vi "CreateQueueName.vi"(0 "VI reference in":refnum<vi> caption="VI reference in (Top-Level)", 11 "Error in":errorcluster caption="Error in (no error)") -> (4 "Queue name":string, 15 "Error out":errorcluster)   [LabVIEW 2017, in "VILauncher.lvlib"]
doc: "Creates the <B>Queue name</B> for the AutoQueue used by the DynamicDispatch toolset.\n\nThis VI is reentrant, and it doesn't run if there is an error on <B>Error in</B>.\n\nSteen Schmidt\nGPower\n26/12 2012"
uses:
  VILauncher.lvlib
panel:
  # "Copyright © 2013\nSteen Schmidt, GPower\nSee enclosed license file for terms and conditions"
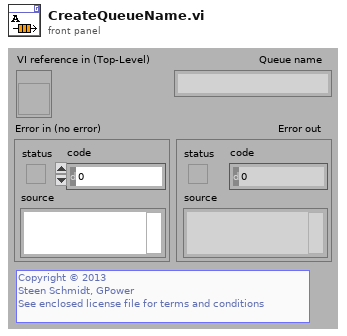
[diagram p1: front panel]
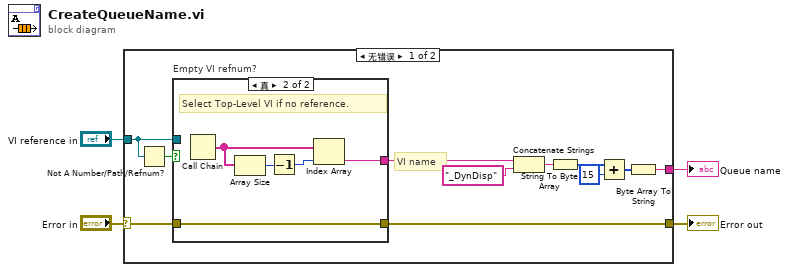
[diagram p0: block diagram]
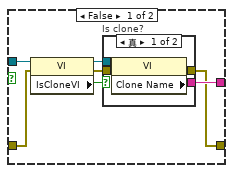
[diagram p2: hidden frame]
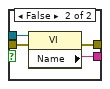
[diagram p3: hidden frame]
diagram:
  n1 = case shown="无错误" "Error in" {
    selector: "Error in" -> [w12 w36]
    tunnel: "VI reference in" -> [w14 _]
    tunnel: [w10 w36] -> w3
    tunnel: [w11 _] -> w1
    frame No Error {
      # "VI name"
      n2 = Not A Number/Path/Refnum?(number/path/refnum=w14) -> (NaN/Path/Refnum?=w15:bool)
      n3 = case "Empty VI refnum?" shown="真" w15 {
        tunnel: w14 -> [w19 _]
        tunnel: w12 -> [w18 w32]
        tunnel: [w17 w31] -> w13
        tunnel: [w16 w32] -> w10
        frame False {
          n4 = property class="VI"(reference=w19, error in=w18) -> (reference out=w21:refnum<vi>, error out=w20:errorcluster, "IsCloneVI"=w22:bool)
          n5 = case "Is clone?" shown="真" w22 {
            tunnel: w20 -> [w26 w30]
            tunnel: w21 -> [w25 w29]
            tunnel: [w24 w28] -> w16
            tunnel: [w23 w27] -> w17
            frame True {
              n6 = property class="VI"(reference=w25, error in=w26) -> (error out=w24:errorcluster, "Clone Name"=w23:string)  [unwired: 1 out]
            }
            frame False {
              n7 = property class="VI"(reference=w29, error in=w30) -> (error out=w28:errorcluster, "Name"=w27:string)  [unwired: 1 out]
            }
          }
        }
        frame True {
          # "Select Top-Level VI if no reference."
          n8 = Call Chain() -> (call chain=w35:string[])
          n9 = Array Size(array=w35) -> (size(s)=w34:i32)
          n10 = Decrement(x=w34) -> (x-1=w33:i32)
          n11 = Index Array(array=w35, index=w33) -> (element=w31:string)
        }
      }
      n12 = Concatenate Strings(w13, "_DynDisp" ("string")) -> (w9:string)
      n13 = String To Byte Array(string=w9) -> (unsigned byte array=w8:u8[])
      n14 = Add(x=w8, y=u8 15) -> (x+y=w6:u8[])
      n15 = Byte Array To String(unsigned byte array=w6) -> (string=w11:string)
    }
    frame Error {
    }
  }
  "Error out" <- w3
  "Queue name" <- w1
